vi "Write Time Flags.vi"(8 "error in (no error)":errorcluster, 10 "Time Flags":T1, 11 "DROPBEAR_Model_Updating in":refnum<class "DROPBEAR_Model_Updating.lvclass">) -> (0 "error out":errorcluster, 3 "DROPBEAR_Model_Updating out":refnum<class "DROPBEAR_Model_Updating.lvclass">)   [LabVIEW 2021, in "DROPBEAR_Model_Updating.lvclass"]
uses:
  DROPBEAR_Model_Updating.lvclass
  DROPBEAR_Model_Updating.lvclass/DROPBEAR_Model_Updating.ctl
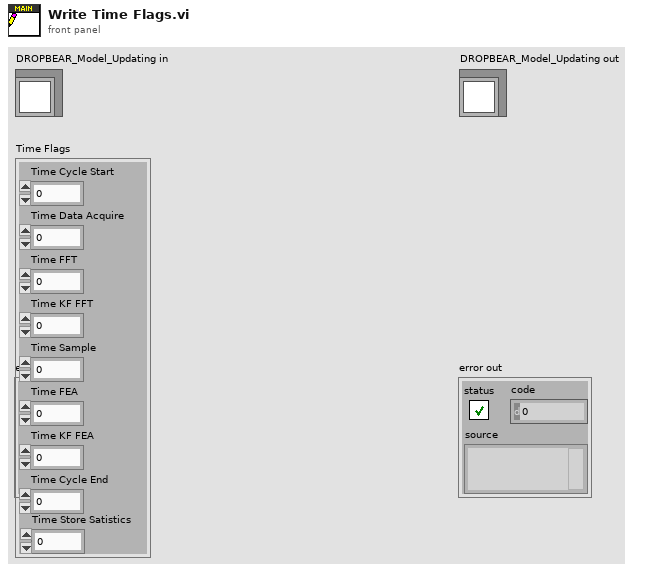
[diagram p1: front panel]
types:
  T1 = cluster{"Time Cycle Start":u32, "Time Data Acquire":u32, "Time FFT":u32, "Time KF FFT":u32, "Time Sample":u32, "Time FEA":u32, "Time KF FEA":u32, "Time Cycle End":u32, "Time Store Satistics":u32}
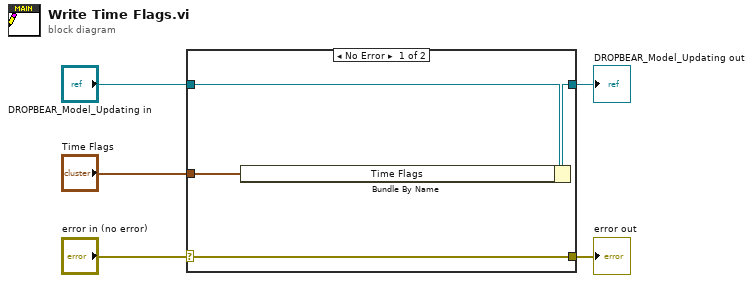
[diagram p0: block diagram]
diagram:
  n1 = case shown="No Error" "error in (no error)" {
    selector: "error in (no error)" -> [w9 w10]
    tunnel: [w9 w10] -> w4
    tunnel: [w7 w11] -> w2
    tunnel: "DROPBEAR_Model_Updating in" -> [w8 w11]
    tunnel: "Time Flags" -> [w6 _]
    frame No Error {
      n2 = Bundle By Name(cluster=w8, "Time Flags"=w6) -> (w7:refnum<class "DROPBEAR_Model_Updating.lvclass">)
    }
    frame Error {
    }
  }
  "error out" <- w4
  "DROPBEAR_Model_Updating out" <- w2
